vi "Load Test Executive.vi"(8 "error in (no error)":errorcluster, 10 "Path":path, 11 "Test Executive Builder Model in":refnum<class "Test Executive Builder Model.lvclass">) -> (0 "error out":errorcluster, 3 "Test Executive Builder Model out":refnum<class "Test Executive Builder Model.lvclass">)   [LabVIEW 2017, in "Test Executive Builder Model.lvclass"]
uses:
  Test Executive Builder Model.lvclass
  <vilib>/gpm_packages/@cs/test-executive/Source/Test Executive/TestExecutive Ref/TestExecutive Ref.lvclass
  Test Executive Builder Model Messages/Redraw Tree Msg/Redraw Tree Msg.lvclass
  <vilib>/ActorFramework/Actor/Actor.lvclass
  <vilib>/gpm_packages/@cs/mva-core/Source/IModel/IModel/IModel.lvclass
  C:/Program Files (x86)/National Instruments/LabVIEW 2017/vi.lib/ActorFramework/Actor/Actor.lvclass
  C:/Users/jonmc/Documents/Git/Test Executive Builder/gpm_packages/@cs/mva-core/Source/IModel/IModel/IModel.lvclass
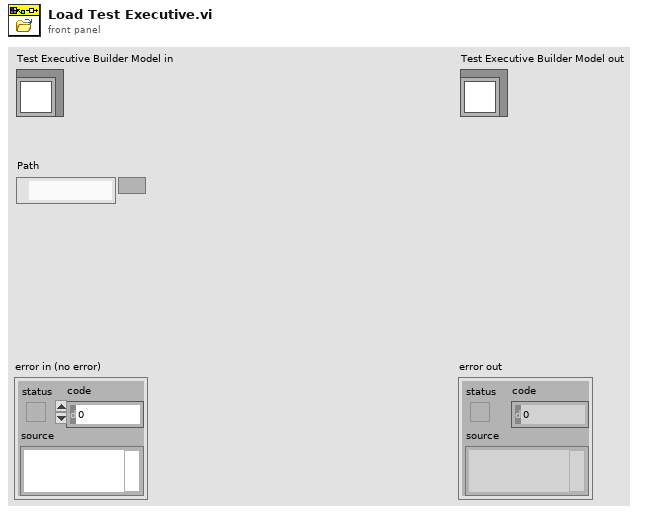
[diagram p1: front panel]
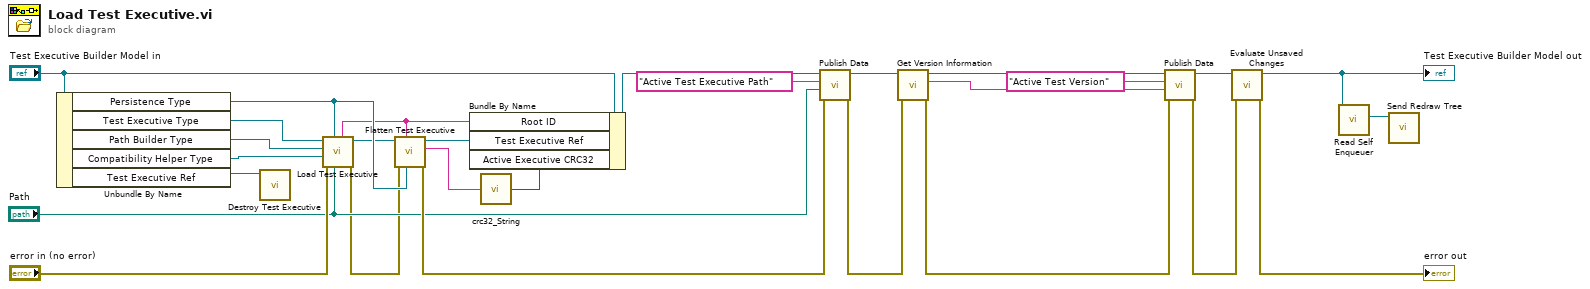
[diagram p0: block diagram]
diagram:
  n1 = Unbundle By Name("Test Executive Builder Model in") -> ("Persistence Type"=w20:refnum<class "IPersist.lvclass">, "Test Executive Type"=w27:refnum<class "ITest Executive.lvclass">, "Path Builder Type"=w23:refnum<class "IPath Builder.lvclass">, "Compatibility Helper Type"=w22:refnum<class "ICompatibility Helper.lvclass">, "Test Executive Ref"=w28:refnum<data-value>)
  n2 = call <vilib>:"Destroy Test Executive.vi"("Test Executive Ref"=w28) -> ()  [unwired: 10 in, 1 out]
  n3 = call <vilib>:"Load Test Executive.vi"("Folder"="Path", "Persistence in"=w20, "error in (no error)"="error in (no error)", "Compatibility Helper"=w22, "Path Builder"=w23, "Test Executive"=w27) -> ("error out"=w6:errorcluster, "Test Executive Ref out"=w7:refnum<data-value>, "Root ID"=w11:string)  [unwired: 3 in]
  n4 = call <vilib>:"Flatten Test Executive.vi"("Persistence in"=w20, "Root ID"=w11, "error in (no error)"=w6, "Test Executive Ref"=w7) -> ("error out"=w14:errorcluster, "Flattened Test Executive"=w19:string, "Test Executive Ref out"=w21:refnum<data-value>)  [unwired: 5 in]
  n5 = call "crc32_String.vi"("String in"=w19) -> ("CRC32"=w18:u32)  [unwired: 1 in]
  n6 = Bundle By Name(cluster="Test Executive Builder Model in", "Root ID"=w11, "Test Executive Ref"=w21, "Active Executive CRC32"=w18) -> (w15:refnum<class "Test Executive Builder Model.lvclass">)
  n7 = call <vilib>:"Publish Data.vi"("error in (no error)"=w14, "Data to Publish"="Path", "Datum Name"="Active Test Executive Path", "IModel in"=w15) -> ("error out"=w3:errorcluster, "IModel out"=w5:refnum<class "Test Executive Builder Model.lvclass">)  [unwired: 6 in]
  n8 = call-dynamic "Get Version Information.vi"("error in (no error)"=w3, "Test Executive Builder Model in"=w5) -> ("error out"=w2:errorcluster, "Version Info"=w1:string, "Test Executive Builder Model out"=w4:refnum<class "Test Executive Builder Model.lvclass">)  [unwired: 7 in]
  n9 = call <vilib>:"Publish Data.vi"("error in (no error)"=w2, "Data to Publish"=w1, "Datum Name"="Active Test Version", "IModel in"=w4) -> ("error out"=w8:errorcluster, "IModel out"=w9:refnum<class "Test Executive Builder Model.lvclass">)  [unwired: 6 in]
  n10 = call-dynamic "Evaluate Unsaved Changes.vi"("error in (no error)"=w8, "Test Executive Builder Model in"=w9) -> ("error out"=→"error out":errorcluster, "Test Executive Builder Model out"=w17:refnum<class "Test Executive Builder Model.lvclass">)  [unwired: 8 in]
  "Test Executive Builder Model out" <- w17
  n11 = call <vilib>:"Read Self Enqueuer.vi"("Actor"=w17) -> ("Self Enqueuer"=w24:refnum<class "Message Enqueuer.lvclass">)  [unwired: 10 in]
  n12 = call "Send Redraw Tree.vi"("Message Enqueuer"=w24) -> ()  [unwired: 9 in, 2 out]
